vi "Pre Launch Init.vi"(11 "Model Base in":refnum<class "Model Base.lvclass">) -> (0 "error out":errorcluster, 3 "Model Base out":refnum<class "Model Base.lvclass">)   [LabVIEW 2023, in "Model Base.lvlib" / "Model Base.lvclass"]
doc: "(<B>Filename</B>: Actor Framework.lvlib:Actor.lvclass:Pre Launch Init.vi)\n\nDefines behavior that occurs after the Launch Nested Actor method is invoked but before the actor's Actor Core method begins running.\n\nBy default, this method does nothing. A descendant class may override it to define behavior."
uses:
  Model Base.lvclass
  Model Base.lvclass/Model Base.ctl
  <vilib>/ActorFramework/Actor/Actor.lvclass
  Interfaces/Incoming Model Base Interface Messages/Initialize Msg/Initialize Msg.lvclass
  C:/Program Files/National Instruments/LabVIEW 2023/vi.lib/ActorFramework/Actor/Actor.lvclass
  C:/Users/bhaghyaraj/Trainings/NI Actor Frameowork/SDLC/Model Base/Model Base/Model Base.lvclass
  C:/Users/bhaghyaraj/Trainings/NI Actor Frameowork/SDLC/Interfaces/Model Base/Incoming Model Base Interface.lvclass
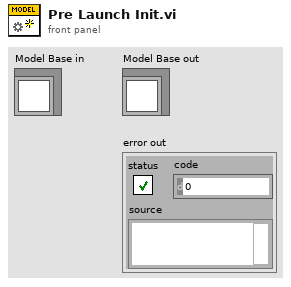
[diagram p1: front panel]
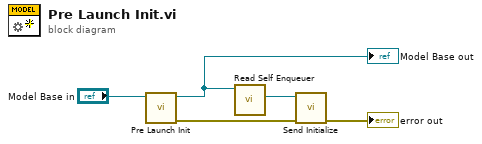
[diagram p0: block diagram]
diagram:
  n1 = call-parent "Pre Launch Init.vi"("Actor in"="Model Base in") -> ("error out"=w5:errorcluster, "Actor out"=w2:refnum<class "Model Base.lvclass">)  [unwired: 9 in]
  "Model Base out" <- w2
  n2 = call <vilib>:"Read Self Enqueuer.vi"("Actor"=w2) -> ("Self Enqueuer"=w1:refnum<class "Message Enqueuer.lvclass">)  [unwired: 10 in]
  n3 = call "Send Initialize.vi"("error in (no error)"=w5, "Message Enqueuer"=w1) -> ("error out"=→"error out":errorcluster)  [unwired: 8 in, 1 out]
